vi "InitializeRequest.vi"(8 "error in (no error)":errorcluster, 10 "Cluster":T1={"option string "="Simulate=1,RangeCheck=1,QueryInstrStatus=0,Cache=1", "id query (Yes)"=TRUE, "reset device (Yes)"=TRUE}, 11 "ModuleID":i32) -> (0 "error out":errorcluster)   [LabVIEW 2018, in "AcPwrPlugins.lvlib" / "AcPwrBase.lvclass"]
uses:
  AcPwrBase.lvclass
  AcPwrModule/Protected/clEventType.ctl
  <vilib>/Utility/error.llb/Error Cluster From Error Code.vi
  <vilib>/ErrorRing/Error Ring.xnode
  AcPwrModule/AcPwrModule.lvlib
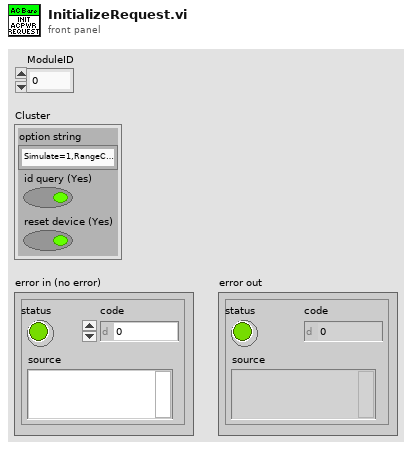
[diagram p1: front panel]
types:
  T1 = cluster{"option string ":string, "id query (Yes)":bool, "reset device (Yes)":bool}
  T2 = typedef "AcPwrModule.lvlib/clRequestEvents.ctl" = cluster{"StopRequest":refnum<user-event>, "PathToINI":refnum<user-event>, " LoadPlugin":refnum<user-event>, "ShowPanel":refnum<user-event>, "PrefDlg":refnum<user-event>, "InitAcPwr":refnum<user-event>, "Reset":refnum<user-event>, "Close":refnum<user-event>, "StopMeas":refnum<user-event>, "StartMeas":refnum<user-event>, "ConfigDevice":refnum<user-event>, "DeviceOn":refnum<user-event>, "DeviceOff":refnum<user-event>}
  T3 = typedef "AcPwrModule.lvlib/clEventType.ctl" = cluster{"ModuleID":i32, "Data":variant}
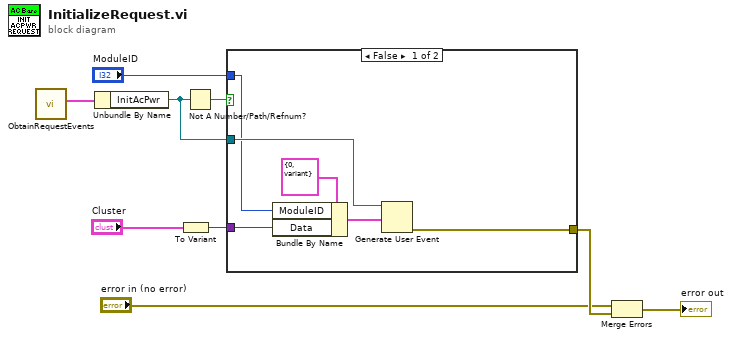
[diagram p0: block diagram]
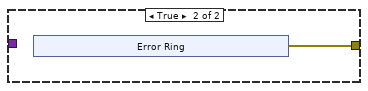
[diagram p2: hidden frame]
diagram:
  n1 = call "ObtainRequestEvents.vi"() -> ("clRequestEvents"=w3:T2)  [unwired: 10 in, 1 out]
  n2 = Unbundle By Name(w3) -> ("InitAcPwr"=w8:refnum<user-event>)
  n3 = To Variant(anything="Cluster") -> (Variant=w1:variant)
  n4 = Not A Number/Path/Refnum?(number/path/refnum=w8) -> (NaN/Path/Refnum?=w9:bool)
  n5 = case shown="False" w9 {
    tunnel: w8 -> [w14 _]
    tunnel: "ModuleID" -> [w12 _]
    tunnel: [w13 w16] -> w5
    tunnel: w1 -> [w10 _]
    frame False {
      n6 = Bundle By Name(cluster=T3 {"ModuleID"=0, "Data"=variant} ("clEventType"), "ModuleID"=w12, "Data"=w10) -> (w15:T3)
      n7 = Generate User Event(user event=w14, event data cluster=w15) -> (error out=w13:errorcluster)  [unwired: 2 in, 1 out]
    }
    frame True {
      n8 = xnode "Error Ring"() -> ("error out"=w16:errorcluster)
    }
  }
  n9 = Merge Errors("error in (no error)", w5) -> (→"error out":errorcluster)
